vi "PR4000B tester.vi"(1 "write buffer":string) -> (0 "read buffer":string)   [LabVIEW 2019]
panel:
  out "error out":errorcluster
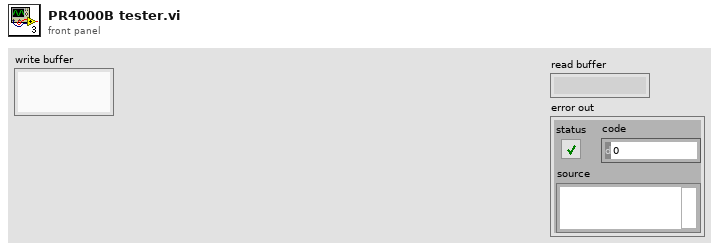
[diagram p1: front panel]
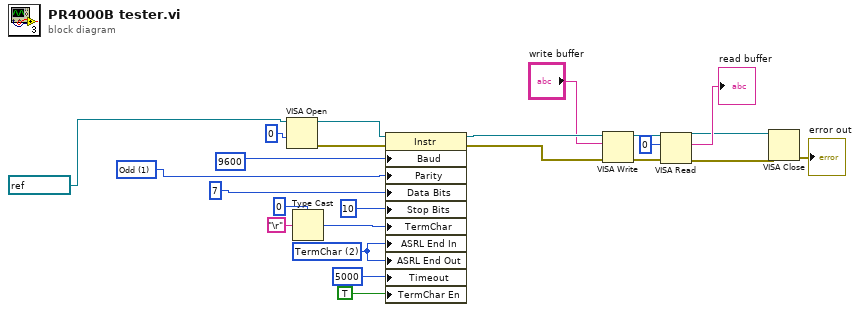
[diagram p0: block diagram]
diagram:
  w2 = u16 1 items=["None", "Odd", "Even", "Mark", "Space"] ("Serial Settings:Parity (Odd)")
  w17 = u16 2 items=["None", "Last Bit", "TermChar"] ("Serial Settings:End Mode for Reads")
  n1 = VISA Open(access mode=u32 0, VISA resource name=refnum<visa-resource-name> "COM5") -> (VISA resource name=w21:refnum<visa-resource-name>, error out=w20:errorcluster)  [unwired: 3 in]
  n2 = Type Cast(type=u8 0, x="\r") -> (*(type *) &x=w18:u8)
  n3 = property class="Instr"(reference=w21, error in=w20, "Baud"=u32 9600 ("Serial Settings:Baud Rate"), "Parity"=w2, "Data Bits"=u16 7 ("Serial Settings:Data Bits (7)"), "Stop Bits"=u16 10 ("ASRL Stop Bits"), "TermChar"=w18, "ASRL End In"=w17, "ASRL End Out"=w17, "Timeout"=u32 5000 ("General Settings:Timeout Value"), "TermChar En"=TRUE ("Message Based Settings:Termination Character Enable")) -> (reference out=w13:refnum<visa-resource-name>, error out=w12:errorcluster)
  n4 = VISA Write(VISA resource name=w13, write buffer="write buffer", error in (no error)=w12) -> (VISA resource name out=w9:refnum<visa-resource-name>, error out=w10:errorcluster)  [unwired: 1 out]
  n5 = VISA Read(VISA resource name=w9, byte count=u32 0, error in (no error)=w10) -> (VISA resource name out=w6:refnum<visa-resource-name>, read buffer=→"read buffer":string, error out=w7:errorcluster)  [unwired: 1 out]
  n6 = VISA Close(VISA resource name=w6, error in (no error)=w7) -> (error out=→"error out":errorcluster)
